vi "niRFUtil MT UTIL Generate Filter Coefficients Validate.vi"(0 "System Filter Characteristic (none)":T2(ring), 1 "Modulation Type":T1(ring), 5 "Modulation Samples Per Symbol (16)":i32=16, 7 "Demodulation Samples Per Symbol (16)":i32=16, 9 "Filter Parameter":dbl=0.5 format="%.2f", 11 "Filter Length (3)":i32=3) -> (15 "error out":errorcluster)   [LabVIEW 2015, in "niRFUtil.lvlib"]
doc: "Validates the inputs for generating filter taps."
uses:
  niRFUtil.lvlib
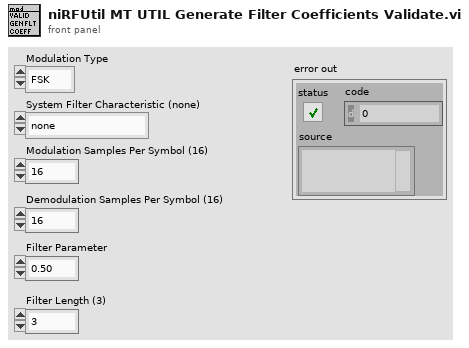
[diagram p1: front panel]
types:
  T1 = enum16{"FSK", "PSK", "QAM", "MSK", "PAM", "ASK", "CPM"}
  T2 = enum16{"none", "Raised Cosine", "Root Raised Cos", "Gaussian"}
  T3 = cluster{"status":bool, "code":i32, "name":string}
  T4 = cluster{"status":bool, "code":i32, "name":string}[]
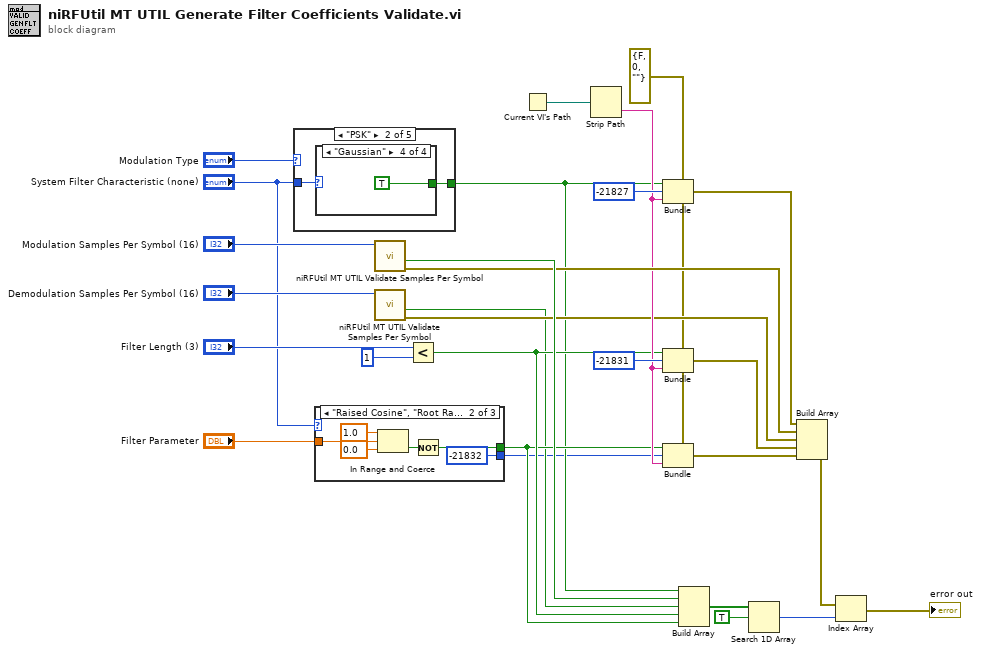
[diagram p0: block diagram]
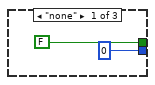
[diagram p2: hidden frame]
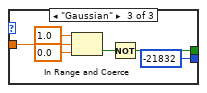
[diagram p3: hidden frame]
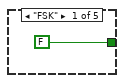
[diagram p4: hidden frame]
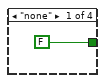
[diagram p5: hidden frame]
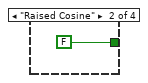
[diagram p6: hidden frame]
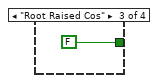
[diagram p7: hidden frame]
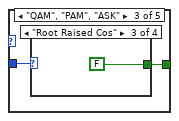
[diagram p8: hidden frame]
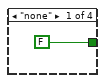
[diagram p9: hidden frame]
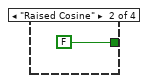
[diagram p10: hidden frame]
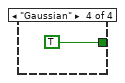
[diagram p11: hidden frame]
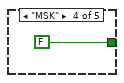
[diagram p12: hidden frame]
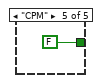
[diagram p13: hidden frame]
diagram:
  w1 = T3 {"status"=FALSE, "code"=0, "name"=""} ("element")
  n1 = case shown="\"PSK\"" "Modulation Type" {
    tunnel: "System Filter Characteristic (none)" -> [_ w31 w37 _ _]
    tunnel: [FALSE ("element") w30 w36 FALSE ("element") FALSE ("element")] -> w4
    frame "FSK" {
    }
    frame "PSK" {
      n2 = case shown="\"Gaussian\"" w31 {
        tunnel: [FALSE ("element") FALSE ("element") FALSE ("element") TRUE ("element")] -> w30
        frame "none" {
        }
        frame "Raised Cosine" {
        }
        frame "Root Raised Cos" {
        }
        frame "Gaussian" {
        }
      }
    }
    frame "QAM", "PAM", "ASK" {
      n3 = case shown="\"Root Raised Cos\"" w37 {
        tunnel: [FALSE ("element") FALSE ("element") FALSE ("element") TRUE ("element")] -> w36
        frame "none" {
        }
        frame "Raised Cosine" {
        }
        frame "Root Raised Cos" {
        }
        frame "Gaussian" {
        }
      }
    }
    frame "MSK" {
    }
    frame "CPM" {
    }
  }
  n4 = case shown="\"Raised Cosine\", \"Root Raised Cos\"" "System Filter Characteristic (none)" {
    tunnel: "Filter Parameter" -> [_ w51 w57]
    tunnel: [FALSE w47 w53] -> w8
    tunnel: [0 ("code") -21832 ("code") -21832 ("code")] -> w2
    frame "none" {
    }
    frame "Raised Cosine", "Root Raised Cos" {
      n5 = In Range and Coerce(upper limit=1.0, x=w51, lower limit=0.0) -> (In Range?=w48:bool)  [unwired: 1 out]
      n6 = Not(x=w48) -> (.not. x?=w47:bool)
    }
    frame "Gaussian" {
      n7 = In Range and Coerce(upper limit=1.0, x=w57, lower limit=0.0) -> (In Range?=w54:bool)  [unwired: 1 out]
      n8 = Not(x=w54) -> (.not. x?=w53:bool)
    }
  }
  n9 = call "niRFUtil MT UTIL Validate Samples Per Symbol.vi"("Samples Per Symbol"="Modulation Samples Per Symbol (16)") -> ("error out"=w14:errorcluster, "error?"=w15:bool)  [unwired: 9 out]
  n10 = call "niRFUtil MT UTIL Validate Samples Per Symbol.vi"("Samples Per Symbol"="Demodulation Samples Per Symbol (16)") -> ("error out"=w5:errorcluster, "error?"=w3:bool)  [unwired: 9 out]
  n11 = Less?(x="Filter Length (3)", y=1) -> (x < y?=w9:bool)
  n12 = Current VI's Path() -> (path=w21:path)
  n13 = Strip Path(path=w21) -> (name=w10:string)  [unwired: 1 out]
  n14 = Bundle(cluster=w1, "status"=w4, "code"=-21827, "name"=w10) -> (w6:T3)
  n15 = Bundle(cluster=w1, "status"=w9, "code"=-21831, "name"=w10) -> (w28:T3)
  n16 = Bundle(cluster=w1, "status"=w8, "code"=w2, "name"=w10) -> (w26:T3)
  n17 = Build Array(w4, w15, w3, w9, w8) -> (w24:bool[])
  n18 = Search 1D Array(1D array=w24, element=TRUE) -> (index of element=w22:i32)  [unwired: 1 out]
  n19 = Build Array(w6, w14, w5, w28, w26) -> (w25:T4)
  n20 = Index Array(array=w25, index=w22) -> (element=→"error out":T3)
